vi "Create_Default_Destinations.vi"(8 "error in (no error)":errorcluster, 9 "Destination Name":string, 10 "Destination Path":path, 11 "AB_DepDLL in":refnum<class "AB_DepDLL.lvclass">) -> (0 "error out":errorcluster, 2 "default dests":refnum<class "AB_Destination.lvclass">[](array[class]), 3 "AB_DepDLL out":refnum<class "AB_DepDLL.lvclass">)   [LabVIEW 2020, in "AB_DepDLL.lvclass"]
uses:
  <vilib>/AppBuilder/AB_Classes/DepDLL/AB_DepDLL.lvclass
  e:/builds/penguin/labview/branches/2020/dev/dist/vi.lib/AppBuilder/AB_Classes/Build/AB_Build.lvclass
  <vilib>/AppBuilder/AB_Classes/Destination/AB_Destination.lvclass
  <vilib>/AppBuilder/AB_Classes/Build/AB_Build.lvclass/AB_Build.ctl
  <vilib>/AppBuilder/AB_Classes/DLL/AB_DLL.lvclass
  <vilib>/AppBuilder/AB_Classes/Build/AB_Build.lvclass
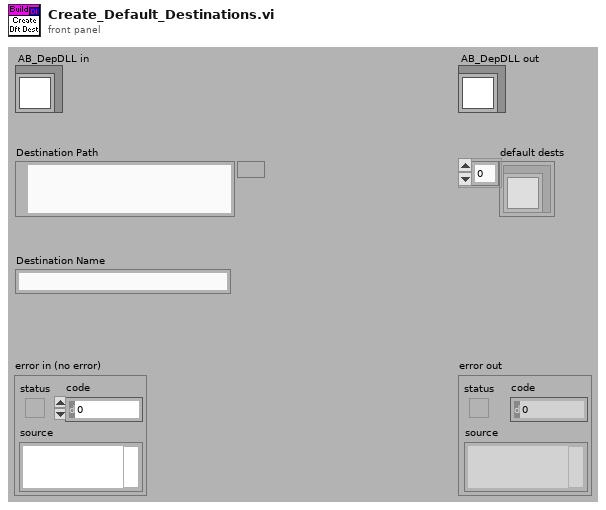
[diagram p1: front panel]
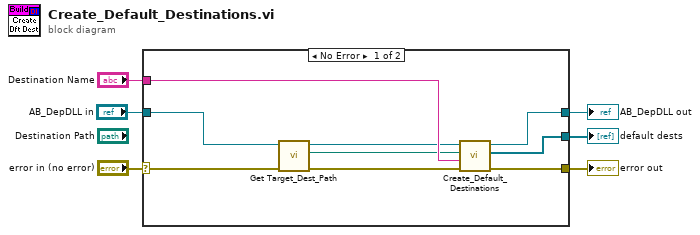
[diagram p0: block diagram]
diagram:
  n1 = case shown="No Error" "error in (no error)" {
    selector: "error in (no error)" -> [w8 w17]
    tunnel: [w15 w17] -> w6
    tunnel: [w14 _] -> w5
    tunnel: [w13 w16] -> w4
    tunnel: "Destination Name" -> [w12 _]
    tunnel: "AB_DepDLL in" -> [w11 w16]
    frame No Error {
      n2 = call <vilib>:"Get Target_Dest_Path.vi"("error in (no error)"=w8, "AB_Build in"=w11) -> ("error out"=w9:errorcluster, "Target Dest Path"=w7:path, "AB_Build out"=w10:refnum<class "AB_DepDLL.lvclass">)  [unwired: 7 in]
      n3 = call-parent "Create_Default_Destinations.vi"("error in (no error)"=w9, "Destination Name"=w12, "Destination Path"=w7, "AB_Application in"=w10) -> ("error out"=w15:errorcluster, "default dests"=w14:refnum<class "AB_Destination.lvclass">[], "AB_Application out"=w13:refnum<class "AB_DepDLL.lvclass">)  [unwired: 5 in]
    }
    frame Error {
    }
  }
  "error out" <- w6
  "AB_DepDLL out" <- w4
  "default dests" <- w5
